vi "workspace_cache.get.vi"(8 "error in":errorcluster, 11 "Nominal Client in":refnum<class "Nominal Client.lvclass">) -> (0 "error out":errorcluster, 2 "Workspace":refnum<class "workspace.lvclass">[](array[class]), 3 "Nominal Client out":refnum<class "Nominal Client.lvclass">)   [LabVIEW 2020, in "Nominal Client.lvclass"]
uses:
  Nominal Client.lvclass
  Nominal Client.lvclass/Nominal Client.ctl
  nominal types/workspace/workspace.lvclass
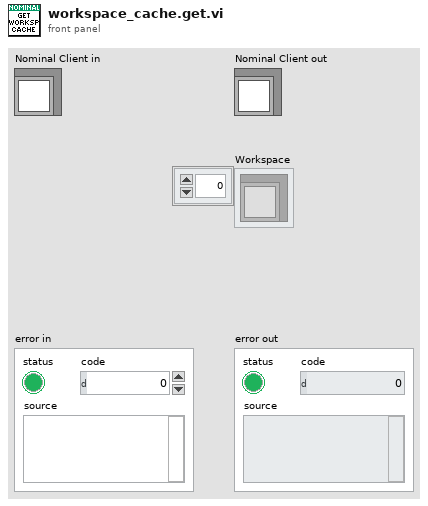
[diagram p1: front panel]
types:
  T1 = typedef "Nominal Client.lvclass/private_data.ctl" = cluster{"API Token":string, "REST Client":refnum<class "REST Client.lvclass">, "workspace":refnum<class "workspace.lvclass">, "Available Workspaces":refnum<class "workspace.lvclass">[]}
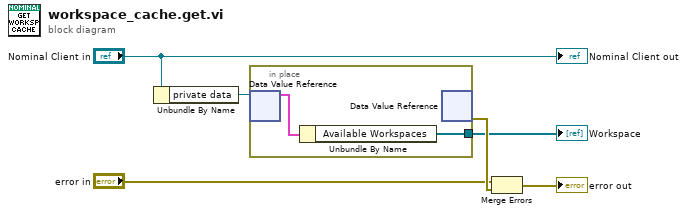
[diagram p0: block diagram]
diagram:
  n1 = Unbundle By Name("Nominal Client in") -> ("private data"=w6:refnum<data-value>)
  n2 = in-place {
    in-place-border: [w7] -> w2
    n3 = in-place-dvr #1(w6) -> (w8:T1)  [unwired: 1 out]
    n4 = Unbundle By Name(w8) -> ("Available Workspaces"=w7:refnum<class "workspace.lvclass">[])
    n5 = in-place-dvr #1() -> (w5:errorcluster)  [unwired: 1 in, 1 out]
  }
  "Workspace" <- w2
  n6 = Merge Errors("error in", w5) -> (→"error out":errorcluster)
  "Nominal Client out" <- "Nominal Client in"
